vi "FileIO_GetCreationDate.vi"(0 "File Path":path, 11 "Error In":errorcluster) -> (4 "File Path 2":path, 6 "Successful":bool, 8 "Time Stamp Control":timestamp, 15 "Error Out":errorcluster)   [LabVIEW 2016]
doc: "Returns the File/Folder creation date for the given path."
uses:
  kernel32.dll
panel:
  in  "date time rec":T1
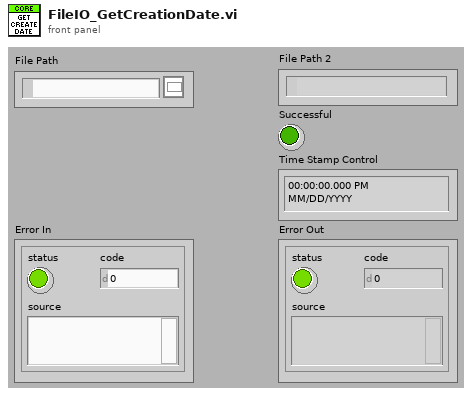
[diagram p1: front panel]
types:
  T1 = cluster{"fractional second":dbl, "second":i32, "minute":i32, "hour":i32, "day of month":i32, "month":i32, "year":i32, "day of week":i32, "day of year":i32, "DST":i32}
  T2 = cluster{"wYear":u16, "wMonth":u16, "wDayOfWeek":u16, "wDay":u16, "wHour":u16, "wMinute":u16, "wSeconds":u16, "wMilliseconds":u16}
  T3 = cluster{"dwFileAttributes":i32, "ftCreationTime":cluster{"dwLowDateTime":i32, "dwHighDateTime":i32}, "ftLastAccessTime":cluster{"dwLowDateTime":i32, "dwHighDateTime":i32}, "ftLastWrittenTime":cluster{"dwLowDateTime":i32, "dwHighDateTime":i32}, "nFileSizeHigh":i32, "nFileSizeLow":i32}
  T4 = cluster{"dwLowDateTime":i32, "dwHighDateTime":i32}
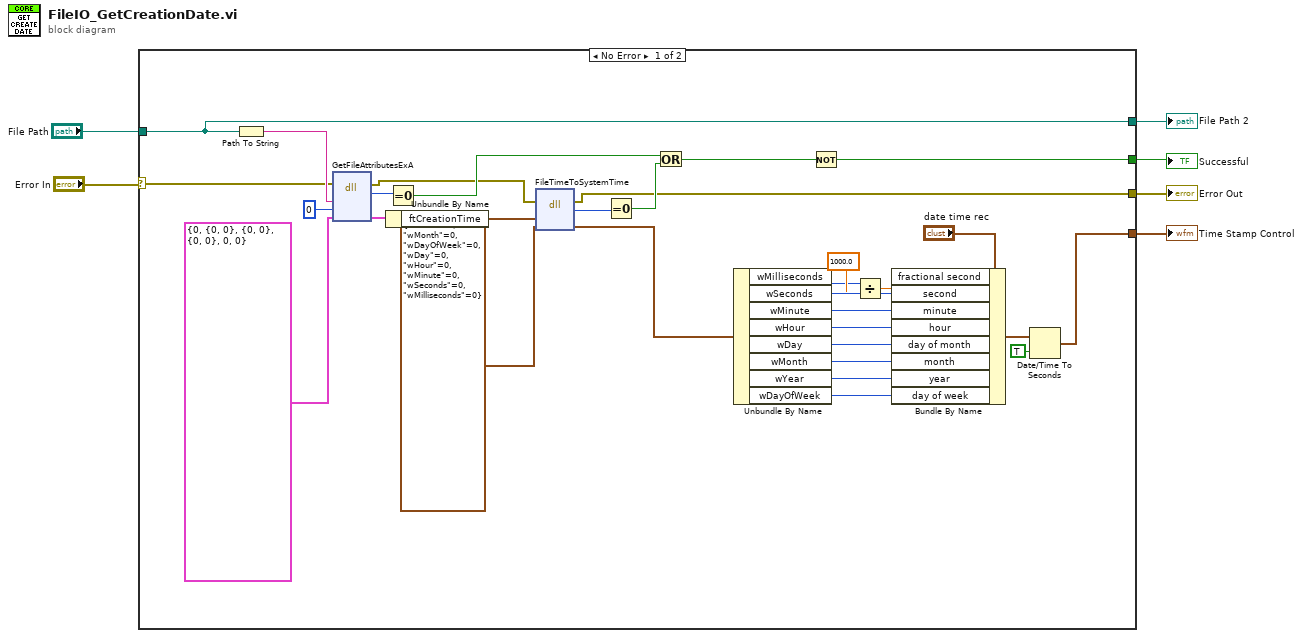
[diagram p0: block diagram]
diagram:
  n1 = case shown="No Error" "Error In" {
    selector: "Error In" -> [w8 w39]
    tunnel: [w13 _] -> w6
    tunnel: [w11 w39] -> w5
    tunnel: [w9 _] -> w4
    tunnel: "File Path" -> [w7 w38]
    tunnel: [w7 w38] -> w1
    frame No Error {
      n2 = Path To String(path=w7) -> (string=w37:string)
      n3 = dll-call lib="kernel32.dll" fn="GetFileAttributesExA" label="GetFileAttributesEx"(error in=w8, "lpFileName"=w37, "fInfoLevelID"=0, "output param"=T3 {"dwFileAttributes"=0, "ftCreationTime"={"dwLowDateTime"=0, "dwHighDateTime"=0}, "ftLastAccessTime"={"dwLowDateTime"=0, "dwHighDateTime"=0}, "ftLastWrittenTime"={"dwLowDateTime"=0, "dwHighDateTime"=0}, "nFileSizeHigh"=0, "nFileSizeLow"=0}) -> (error out=w12:errorcluster, w31:i32, "output param"=w34:T3)  [unwired: 4 in, 1 out]
      n4 = Unbundle By Name(w34) -> ("ftCreationTime"=w33:T4)
      n5 = Equal To 0?(x=w31) -> (x = 0?=w28:bool)
      n6 = dll-call lib="kernel32.dll" fn="FileTimeToSystemTime"(error in=w12, "ftCreationTime"=w33, "output param"=T2 {"wYear"=0, "wMonth"=0, "wDayOfWeek"=0, "wDay"=0, "wHour"=0, "wMinute"=0, "wSeconds"=0, "wMilliseconds"=0}) -> (error out=w11:errorcluster, w30:i32, "output param"=w26:T2)  [unwired: 3 in, 1 out]
      n7 = Equal To 0?(x=w30) -> (x = 0?=w29:bool)
      n8 = Or(x=w28, y=w29) -> (x .or. y?=w27:bool)
      n9 = Unbundle By Name(w26) -> ("wMilliseconds"=w16:u16, "wSeconds"=w25:u16, "wMinute"=w24:u16, "wHour"=w23:u16, "wDay"=w22:u16, "wMonth"=w21:u16, "wYear"=w20:u16, "wDayOfWeek"=w19:u16)
      n10 = Not(x=w27) -> (.not. x?=w9:bool)
      n11 = Divide(x=w16, y=1000.0) -> (x/y=w15:dbl)
      n12 = Bundle By Name(cluster="date time rec", "fractional second"=w15, "second"=w25, "minute"=w24, "hour"=w23, "day of month"=w22, "month"=w21, "year"=w20, "day of week"=w19) -> (w14:T1)
      n13 = Date/Time To Seconds(1:TRUE ("is UTC (F)"), 2:w14) -> (0:w13:timestamp)
    }
    frame Error {
    }
  }
  "Time Stamp Control" <- w6
  "Error Out" <- w5
  "Successful" <- w4
  "File Path 2" <- w1
